vi "myRIO_BRig_RT_dataMTrig_Solenoid_Tdelay__L.vi"() -> (2 "output_Solenoid_Tdelay__L":i32)   [LabVIEW 2014]
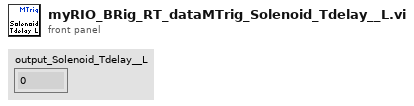
[diagram p1: front panel]
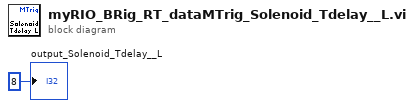
[diagram p0: block diagram]
diagram:
  "output_Solenoid_Tdelay__L" <- 8 ("output_iBlock")
